vi "FTW-FileSystem-FileVersion.vi"(11 "error in":errorcluster) -> (4 "Version":string, 15 "error out":errorcluster)   [LabVIEW 2013]
panel:
  # "Inputs"
  # "Outputs"
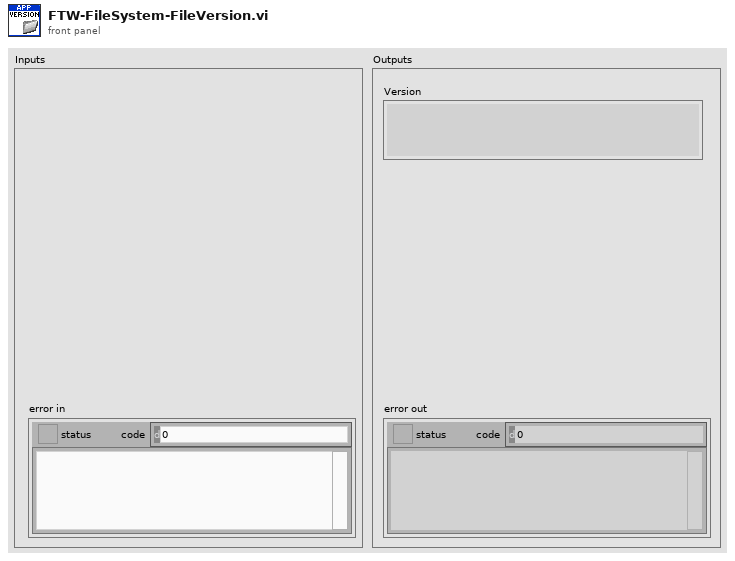
[diagram p1: front panel]
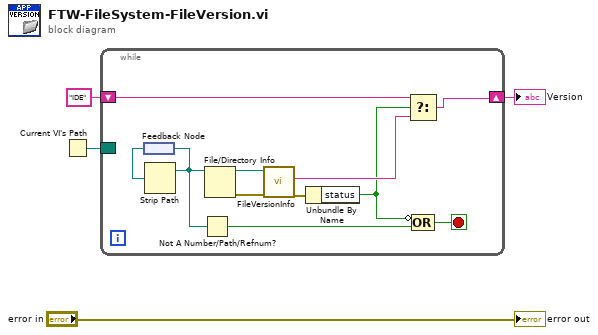
[diagram p0: block diagram]
diagram:
  n1 = Current VI's Path() -> (path=w2:path)
  n2 = while {
    border: w2 -> [_]
    shift-right: [w8] -> w1
    shift-left: "IDE" ("File Version Info") -> [w9]
    stop <- w10 stop-if-true
    n3 = feedback #1() -> (w13:path)
    n4 = Strip Path(path=w13) -> (stripped path=w12:path)  [unwired: 1 out]
    n5 = feedback-in #1(w12) -> ()
    n6 = Not A Number/Path/Refnum?(number/path/refnum=w12) -> (NaN/Path/Refnum?=w11:bool)
    n7 = File/Directory Info(path=w12) -> (path out=w14:path, error out=w15:errorcluster)  [unwired: 1 in, 5 out]
    n8 = call <vilib>:"FileVersionInfo.vi"("error in (no error)"=w15, "Application Path in"=w14) -> ("error out"=w6:errorcluster, "File Version Info"=w7:string)  [unwired: 6 in, 2 out]
    n9 = Unbundle By Name(w6) -> ("status"=w5:bool)
    n10 = Select(t=w9, s=w5, f=w7) -> (s? t:f=w8:string)
    n11 = Compound Arithmetic op=OR(invert w5, w11) -> (w10:bool)
  }
  "Version" <- w1
  "error out" <- "error in"
